vi "Fluke 28x Series Arbitrary Waveform Sequence.vi"() -> ()   [LabVIEW 2015]
doc: "This example shows how to configure a sequence of arbitrary waveforms."
uses:
  Instance           1 52Saved   Fluke 28x Series Arbitrary Waveform Sequence .vi
  Instance           2 52Saved   Fluke 28x Series Arbitrary Waveform Sequence .vi
  <instrlib>/Fluke 28x Series/Fluke 28x Series.lvlib
panel:
  in  "Arbitrary Waveform Name":string[](array[string])
  in  "Enable Sequence Segment (T: Enable)":bool[](array[boolean])=[TRUE]
  in  "Start Sequence Step (Count)":u16[](array[ring]) items=["Count", "Trigger Edge", "Trigger Level"]
  in  "Sequence Iterations (1)":dbl[](array[numeric]) min=1.0 max=32768.0
  in  "VISA resource name":refnum<visa-resource-name>
  # "(c) 2009-2014 National Instruments.  ALL RIGHTS RESERVED."
  # "This example both allows the user to create several waveforms as well as use\nthese waveforms in the Sequence."
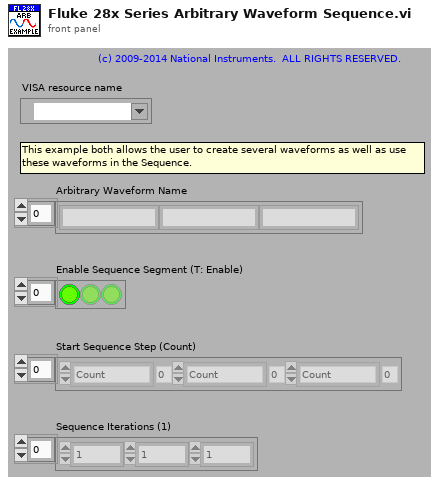
[diagram p1: front panel]
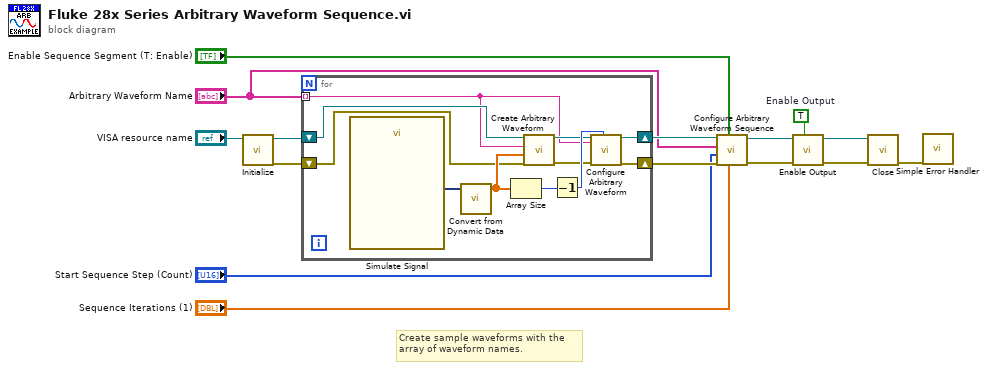
[diagram p0: block diagram]
diagram:
  w1 = TRUE  # Enable Output
  # "Create sample waveforms with the\narray of waveform names."
  n1 = call <instrlib>:"Initialize.vi"("VISA resource name"="VISA resource name") -> ("error out"=w13:errorcluster, "VISA resource name out"=w14:refnum<visa-resource-name>)  [unwired: 9 in]
  n2 = for {
    shift-right: [w23] -> w12
    shift-left: w14 -> [w19]
    shift-right: [w20] -> w11
    shift-left: w13 -> [w18]
    tunnel: "Arbitrary Waveform Name" -> [w17] mode=indexing
    n3 = call "Simulate Signal"() -> ("Triangle"=w26:dynamicdata)  [unwired: 14 in, 1 out]
    n4 = call "Convert from Dynamic Data"("Dynamic Data Type"=w26) -> ("Array"=w25:dbl[])  [unwired: 3 in]
    n5 = Array Size(array=w25) -> (size(s)=w16:i32)
    n6 = call <instrlib>:"Create Arbitrary Waveform.vi"("error in (no error)"=w18, "Arbitrary Waveform Data"=w25, "Arbitrary Waveform Name"=w17, "VISA resource name"=w19) -> ("error out"=w21:errorcluster, "VISA resource name out"=w22:refnum<visa-resource-name>)  [unwired: 6 in]
    n7 = Decrement(x=w16) -> (x-1=w24:i32)
    n8 = call <instrlib>:"Configure Arbitrary Waveform.vi"("VISA resource name"=w22, "Arbitrary Waveform Name"=w17, "error in (no error)"=w21, "Line Stop Address"=w24) -> ("VISA resource name out"=w23:refnum<visa-resource-name>, "error out"=w20:errorcluster)  [unwired: 14 in]
  }
  n9 = call <instrlib>:"Configure Arbitrary Waveform Sequence.vi"("Sequence Iterations (1)"="Sequence Iterations (1)", "Enable Sequence Segment (T: Enable)"="Enable Sequence Segment (T: Enable)", "error in (no error)"=w11, "Start Sequence Step (0: Count)"="Start Sequence Step (Count)", "Arbitrary Sequence Waveform Name"="Arbitrary Waveform Name", "VISA resource name"=w12) -> ("error out"=w4:errorcluster, "VISA resource name out"=w5:refnum<visa-resource-name>)  [unwired: 4 in]
  n10 = call <instrlib>:"Enable Output.vi"("Enable Output (T: Enable)"=w1, "error in (no error)"=w4, "VISA resource name"=w5) -> ("error out"=w2:errorcluster, "VISA resource name out"=w3:refnum<visa-resource-name>)  [unwired: 7 in]
  n11 = call <instrlib>:"Close.vi"("error in (no error)"=w2, "VISA resource name"=w3) -> ("error out"=w9:errorcluster)  [unwired: 9 in]
  n12 = call <vilib>:"Simple Error Handler.vi"("error in (no error)"=w9) -> ()  [unwired: 4 in, 5 out]
